vi "Reset P2P stream.vi"(7 "single shot":bool, 11 "scope params":T1={"scope mode"=enum."Stopped", "ticker"=refnum, "samples per simulated"=0, "FPGA ref"=refnum, "P2P params"={"instrument handle"="", "stream session"=refnum, "scale"={"offset"=0.0, "gain"=0.0, "reserved 1"=0.0, "reserved 2"=0.0}, "actual sample rate"=10000000.0, "Trigger"=enum."PFI 0", "SCOPE Resource"="Dev1", "input impedance"=0}, "data mode"=enum."Real IO"} {"P2P params"."input impedance" items=["1 mega ohm"=0, "50 ohms"=2]; "P2P params"."actual sample rate" format="%.2p"}) -> (0 "error out":errorcluster, 3 "scope params out":T1={"scope mode"=enum."Stopped", "ticker"=refnum, "samples per simulated"=0, "FPGA ref"=refnum, "P2P params"={"instrument handle"="", "stream session"=refnum, "scale"={"offset"=0.0, "gain"=0.0, "reserved 1"=0.0, "reserved 2"=0.0}, "actual sample rate"=10000000.0, "Trigger"=enum."PFI 0", "SCOPE Resource"="Dev1", "input impedance"=0}, "data mode"=enum."Real IO"} {"P2P params"."input impedance" items=["1 mega ohm"=0, "50 ohms"=2]; "P2P params"."actual sample rate" format="%.2p"})   [LabVIEW 2013]
uses:
  controls/scope_params.ctl
  Utilities/Ticker/Ticker.lvclass
  controls/ScopeMode.ctl
  Config/FPGAref.ctl
  P2P params.ctl
  trigger_source.ctl
  FPGA/DataMode.ctl
  <instrlib>/niScope/Controls/niScope vertical coupling.ctl
  <instrlib>/niScope/Controls/niScope trigger slope.ctl
  <instrlib>/niScope/Controls/niScope trigger source digital.ctl
  <instrlib>/niScope/Acquire/niScope Get Scaling Coefficients.vi
  <vilib>/FPGAPlugInAG/Dynamic/niLvFpga_P2PGetEndpoint_Dynamic.vi
  <instrlib>/niScope/Configure/Trigger/niScope Configure Trigger Software.vi
  <instrlib>/niScope/Configure/Trigger/niScope Configure Trigger Digital.vi
  <vilib>/rvi/interface/nirviMethod/nirviMethod.xnode
  <vilib>/rvi/errors/niLvFpgaMergeErrorWithErrorCode.vi
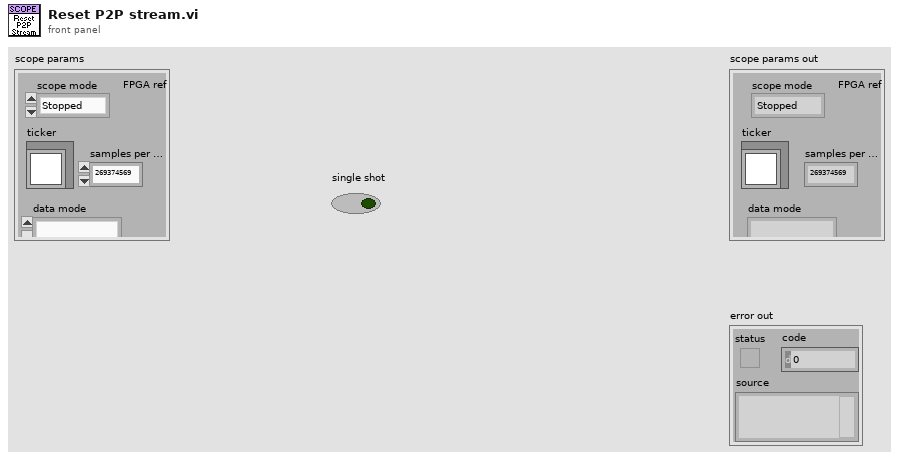
[diagram p1: front panel]
types:
  T1 = typedef "scope_params.ctl" = cluster{"scope mode":T2, "ticker":refnum<class "Ticker.lvclass">, "samples per simulated":u32, "FPGA ref":T3, "P2P params":T4, "data mode":T6}
  T2 = typedef "ScopeMode.ctl" = enum16{"Stopped", "Single", "Running"}
  T3 = typedef "FPGAref.ctl" = refnum<k20>
  T4 = typedef "P2P params.ctl" = cluster{"instrument handle":refnum<k15>, "stream session":refnum<k20>, "scale":cluster{"offset":dbl, "gain":dbl, "reserved 1":dbl, "reserved 2":dbl}, "actual sample rate":dbl, "Trigger":T5, "SCOPE Resource":refnum<k15>, "input impedance":u32}
  T5 = typedef "trigger_source.ctl" = enum16{"PFI 0", "PFI 1", "Software"}
  T6 = typedef "DataMode.ctl" = enum16{"Real IO", "Simulated"}
  T7 = typedef "niScope vertical coupling.ctl" = i32
  T8 = cluster{"offset":dbl, "gain":dbl, "reserved 1":dbl, "reserved 2":dbl}[]
  T9 = cluster{"coefficient info[0]":cluster{"offset":dbl, "gain":dbl, "reserved 1":dbl, "reserved 2":dbl}, "coefficient info[1]":cluster{"offset":dbl, "gain":dbl, "reserved 1":dbl, "reserved 2":dbl}, "coefficient info[2]":cluster{"offset":dbl, "gain":dbl, "reserved 1":dbl, "reserved 2":dbl}, "coefficient info[3]":cluster{"offset":dbl, "gain":dbl, "reserved 1":dbl, "reserved 2":dbl}, "coefficient info[4]":cluster{"offset":dbl, "gain":dbl, "reserved 1":dbl, "reserved 2":dbl}, "coefficient info[5]":cluster{"offset":dbl, "gain":dbl, "reserved 1":dbl, "reserved 2":dbl}, "coefficient info[6]":cluster{"offset":dbl, "gain":dbl, "reserved 1":dbl, "reserved 2":dbl}, "coefficient info[7]":cluster{"offset":dbl, "gain":dbl, "reserved 1":dbl, "reserved 2":dbl}, "coefficient info[8]":cluster{"offset":dbl, "gain":dbl, "reserved 1":dbl, "reserved 2":dbl}}
  T10 = typedef "niScope trigger source digital.ctl" = string
  T11 = typedef "niScope trigger slope.ctl" = i32
  T12 = cluster{"offset":dbl, "gain":dbl, "reserved 1":dbl, "reserved 2":dbl}
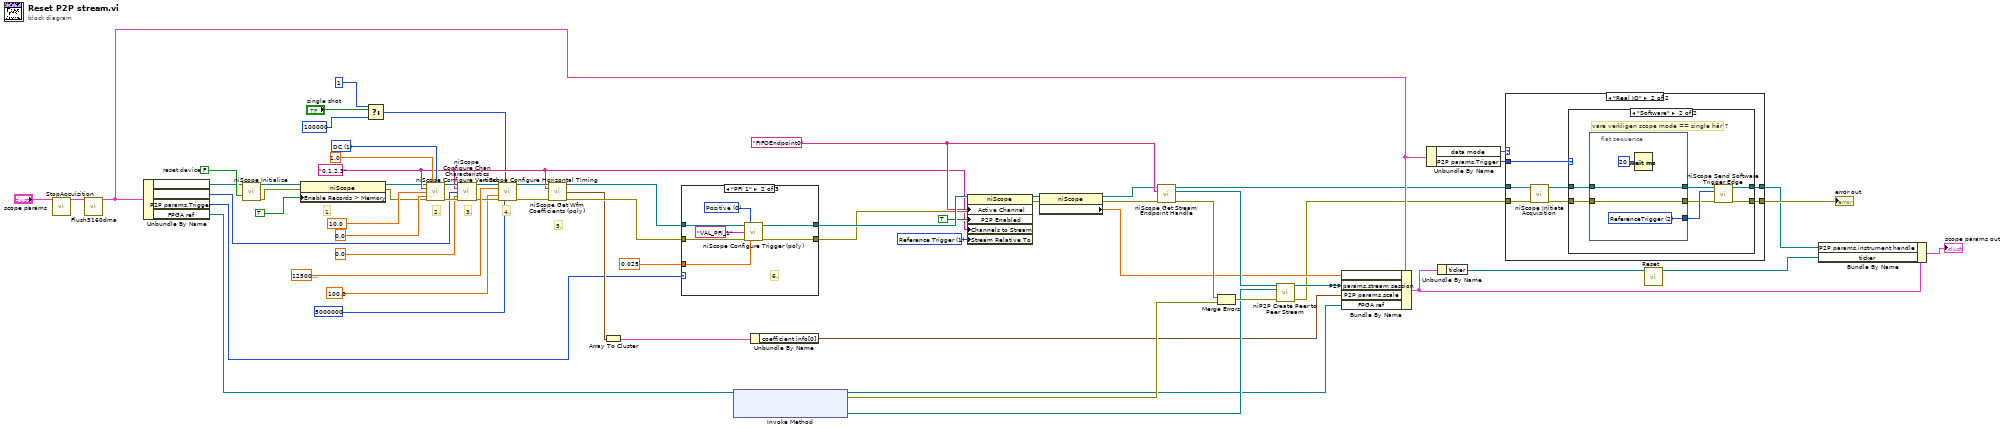
[diagram p0: block diagram]
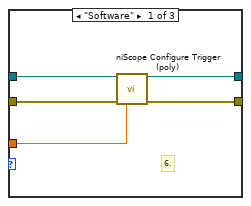
[diagram p4: hidden frame]
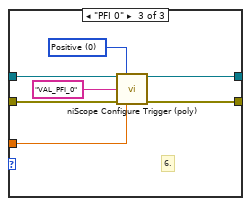
[diagram p5: hidden frame]
diagram:
  w31 = 1 items=["Start Trigger", "Reference Trigger", "Sync Trigger"] ("Peer-to-Peer:Stream Relative To")
  w55 = T7 1 items=["AC", "DC", "Ground"] ("vertical coupling")
  w45 = "0,1,2,3" ("channel name")
  w51 = "FIFOEndpoint0" ("Active Channel")
  w65 = FALSE  # reset device
  # "5."
  # "4."
  # "3."
  # "2."
  # "1."
  n1 = call "StopAqcuisition.vi"("scope in"="scope params") -> ("scope out"=w17:T1)  [unwired: 9 in, 1 out]
  n2 = call "Flush5160dma.vi"("scope params"=w17) -> ("scope params"=w5:T1)  [unwired: 10 in]
  n3 = Unbundle By Name(w5) -> ("P2P params.SCOPE Resource"=w18:refnum<k15>, "P2P params.input impedance"=w15:u32, "P2P params.Trigger"=w16:T5, "FPGA ref"=w14:T3)
  n4 = call <instrlib>:"niScope Initialize.vi"("resource name"=w18, "reset device"=w65) -> ("instrument handle"=w28:refnum<k15>, "error out"=w26:errorcluster)  [unwired: 12 in]
  n5 = property class="niScope"(reference=w28, error in=w26, "Enable Records > Memory"=TRUE ("Horizontal:Enable Records > Memory")) -> (reference out=w27:refnum<k15>, error out=w25:errorcluster)
  n6 = Select(t=1, s="single shot", f=100000 ("number of records")) -> (s? t:f=w21:i32)
  n7 = call <instrlib>:"niScope Configure Vertical.vi"("instrument handle"=w27, "probe attenuation"=1.0, "vertical coupling"=w55, "channels"=w45, "vertical range"=10.0, "vertical offset"=0.0, "error in"=w25) -> ("instrument handle out"=w62:refnum<k15>, "error out"=w61:errorcluster)  [unwired: 7 in]
  n8 = call <instrlib>:"niScope Configure Chan Characteristics.vi"("instrument handle"=w62, "channels"=w45, "input impedance"=w15, "maximum input frequency"=0.0, "error in"=w61) -> ("instrument handle out"=w59:refnum<k15>, "error out"=w60:errorcluster)  [unwired: 9 in]
  n9 = call <instrlib>:"niScope Configure Horizontal Timing.vi"("instrument handle"=w59, "number of records"=w21, "min sample rate"=1250000000.0, "reference position"=100.0, "error in"=w60, "min record length"=5000000) -> ("instrument handle out"=w49:refnum<k15>, "error out"=w48:errorcluster)  [unwired: 8 in]
  n10 = call-poly <instrlib>:"niScope Get Wfm Coefficients (poly).vi"("instrument handle"=w49, "channels"=w45, "error in"=w48) -> ("instrument handle out"=w47:refnum<k15>, "coefficient info"=w44:T8, "error out"=w46:errorcluster)  [unwired: 10 in]
  n11 = Array To Cluster(array=w44) -> (cluster=w43:T9)
  n12 = case shown="\"PFI 1\"" w16 {
    tunnel: [w70 w77 w84] -> w54
    tunnel: [w69 w76 w83] -> w53
    tunnel: w47 -> [w68 w75 w82]
    tunnel: w46 -> [w67 w74 w81]
    tunnel: 0.025 ("trigger holdoff") -> [w66 w73 w80]
    frame "Software" {
      # "6."
      n13 = call-poly <instrlib>:"niScope Configure Trigger (poly).vi"("instrument handle"=w68, "error in"=w67, "trigger holdoff"=w66) -> ("instrument handle out"=w70:refnum<k15>, "error out"=w69:errorcluster)  [unwired: 11 in]
    }
    frame "PFI 1" {
      w72 = T11 0 items=["Positive", "Negative"] ("trigger slope")
      # "6."
      n14 = call-poly <instrlib>:"niScope Configure Trigger (poly).vi"("instrument handle"=w75, "trigger slope"=w72, "trigger source"=T10 "VAL_PFI_1", "error in"=w74, "trigger holdoff"=w73) -> ("instrument handle out"=w77:refnum<k15>, "error out"=w76:errorcluster)  [unwired: 9 in]
    }
    frame "PFI 0" {
      w79 = T11 0 items=["Positive", "Negative"] ("trigger slope")
      # "6."
      n15 = call-poly <instrlib>:"niScope Configure Trigger (poly).vi"("instrument handle"=w82, "trigger slope"=w79, "trigger source"=T10 "VAL_PFI_0", "error in"=w81, "trigger holdoff"=w80) -> ("instrument handle out"=w84:refnum<k15>, "error out"=w83:errorcluster)  [unwired: 9 in]
    }
  }
  n16 = xnode "Invoke Method"("FPGA VI Reference In"=w14) -> ("FPGA VI Reference Out"=w13:T3, "error out"=w35:errorcluster, "Reader"=w36:refnum<k20>)  [unwired: 1 in]
  n17 = Unbundle By Name(w43) -> ("coefficient info[0]"=w33:T12)
  n18 = property class="niScope"(reference=w54, error in=w53, "Active Channel"=w51, "P2P Enabled"=TRUE ("Peer-to-Peer:P2P Enabled"), "Channels to Stream"=w45, "Stream Relative To"=w31) -> (reference out=w40:refnum<k15>, error out=w39:errorcluster)
  n19 = property class="niScope"(reference=w40, error in=w39) -> (reference out=w37:refnum<k15>, error out=w38:errorcluster, "Horizontal:Actual Sample Rate"=w12:dbl)
  n20 = call <instrlib>:"niScope Get Stream Endpoint Handle.vi"("instrument handle"=w37, "stream endpoint"=w51, "error in"=w38) -> ("instrument handle out"=w3:refnum<k15>, "writer handle"=w50:refnum<k20>, "error out"=w41:errorcluster)  [unwired: 10 in]
  n21 = Merge Errors(w41, w35) -> (w42:errorcluster)
  n22 = call <vilib>:"niP2P Create Peer to Peer Stream.vi"("writer"=w50, "reader"=w36, "error in (no error)"=w42) -> ("stream session"=w34:refnum<k20>, "error out"=w2:errorcluster)  [unwired: 11 in]
  n23 = Bundle By Name(cluster=w5, "P2P params.actual sample rate"=w12, "P2P params.stream session"=w34, "P2P params.scale"=w33, "FPGA ref"=w13) -> (w10:T1)
  n24 = Unbundle By Name(w5) -> ("data mode"=w4:T6, "P2P params.Trigger"=w1:T5)
  n25 = Unbundle By Name(w10) -> ("ticker"=w7:refnum<class "Ticker.lvclass">)
  n26 = case shown="\"Real IO\"" w4 {
    tunnel: w3 -> [w86 w91]
    tunnel: w2 -> [w85 w89]
    tunnel: [w85 w93] -> w11
    tunnel: [w86 w92] -> w9
    tunnel: w1 -> [_ w87]
    frame "Simulated" {
    }
    frame "Real IO" {
      n27 = call <instrlib>:"niScope Initiate Acquisition.vi"("instrument handle"=w91, "error in"=w89) -> ("instrument handle out"=w90:refnum<k15>, "error out"=w88:errorcluster)  [unwired: 12 in]
      n28 = case shown="\"Software\"" w87 {
        tunnel: w90 -> [w95 w100]
        tunnel: [w95 w99] -> w92
        tunnel: w88 -> [w94 w98]
        tunnel: [w94 w96] -> w93
        frame "PFI 0", Default {
        }
        frame "Software" {
          # "vare verkligen scope mode == single här`?"
          n29 = flat-sequence {
            tunnel: [w106] -> w102
            tunnel: [w104] -> w101
            tunnel: w100 -> [w104]
            tunnel: w98 -> [w103]
            tunnel: [w103] -> w97
            frame #0 {
              w106 = u16 2 items=["StartTrigger", "ArmReferenceTrigger", "ReferenceTrigger", "AdvanceTrigger"] ("which trigger")
              n30 = Wait (ms)(milliseconds to wait=u32 20) -> ()  [unwired: 1 out]
            }
          }
          n31 = call <instrlib>:"niScope Send Software Trigger Edge.vi"("instrument handle"=w101, "which trigger"=w102, "error in"=w97) -> ("instrument handle out"=w99:refnum<k15>, "error out"=w96:errorcluster)  [unwired: 11 in]
        }
      }
    }
  }
  "error out" <- w11
  n32 = call "Reset.vi"("Ticker in"=w7) -> ("Ticker out"=w6:refnum<class "Ticker.lvclass">)  [unwired: 9 in, 1 out]
  n33 = Bundle By Name(cluster=w10, "P2P params.instrument handle"=w9, "ticker"=w6) -> (→"scope params out":T1)
